vi "Get Period.vi"(3 "(WavBuf)":refnum<class "(WavBuf).lvclass">) -> (1 "Dt Out":dbl)   [LabVIEW 2016, in "(WavBuf).lvclass"]
uses:
  (WavBuf).lvclass
  (WavBuf).lvclass/(WavBuf).ctl
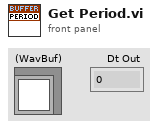
[diagram p1: front panel]
types:
  T1 = typedef "Ref_DVR_Buffer.ctl" = refnum<data-value>
  T2 = typedef "Waveform_Data.ctl" = waveform(dbl)
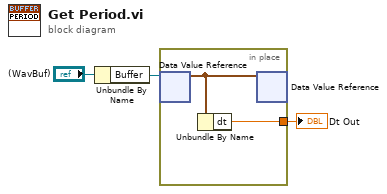
[diagram p0: block diagram]
diagram:
  n1 = Unbundle By Name("(WavBuf)") -> ("Buffer"=w2:T1)
  n2 = in-place {
    in-place-border: [w4] -> w1
    n3 = in-place-dvr #1(w2) -> (w5:T2)  [unwired: 1 out]
    n4 = Unbundle By Name(w5) -> ("dt"=w4:dbl)
    n5 = in-place-dvr #1(w5) -> ()  [unwired: 2 out]
  }
  "Dt Out" <- w1
